vi "Add cod na fila.vi"(2 "error in (no error)":errorcluster, 3 "Queue in":refnum<queue>, 4 "Limite vertical":u32, 5 "Array Cluster in":T1(array[cluster])) -> (0 "error out":errorcluster, 1 "Array Cluster out":T1(array[cluster]))   [LabVIEW 2020]
uses:
  Type Defs/Cluster de envio.ctl
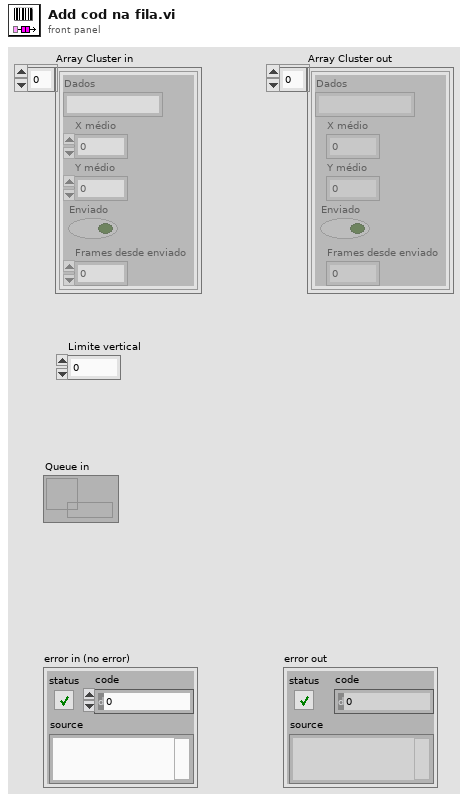
[diagram p1: front panel]
types:
  T1 = cluster{"Dados":string, "X médio":dbl, "Y médio":dbl, "Enviado":bool, "Frames desde enviado":dbl}[]
  T2 = typedef "Cluster de envio.ctl" = cluster{"Código de barras":string, "Quantidade":i32, "Data/Hora":timestamp}
  T3 = cluster{"Dados":string, "X médio":dbl, "Y médio":dbl, "Enviado":bool, "Frames desde enviado":dbl}
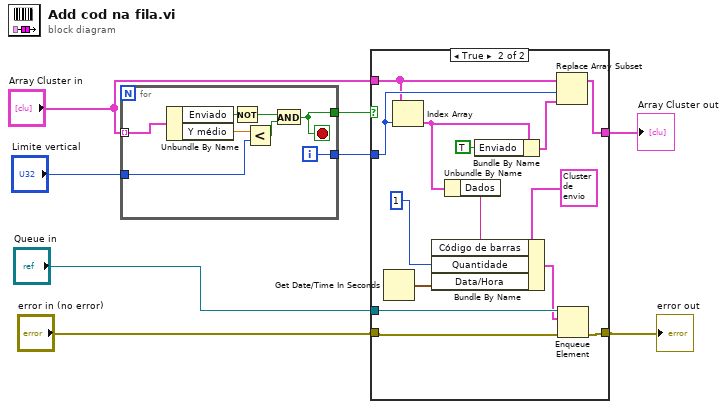
[diagram p0: block diagram]
diagram:
  n1 = for {
    tunnel: "Array Cluster in" -> [w16] mode=indexing
    tunnel: [w14] -> w2
    tunnel: [w10] -> w3
    tunnel: "Limite vertical" -> [w9]
    i -> [w14]
    stop <- w10 stop-if-true
    n2 = Unbundle By Name(w16) -> ("Enviado"=w12:bool, "Y médio"=w15:dbl)
    n3 = Not(x=w12) -> (.not. x?=w13:bool)
    n4 = Less?(x=w15, y=w9) -> (x < y?=w11:bool)
    n5 = And(x=w13, y=w11) -> (x .and. y?=w10:bool)
  }
  n6 = case shown="True" w3 {
    tunnel: "Array Cluster in" -> [w18 w23]
    tunnel: [w18 w25] -> w1
    tunnel: w2 -> [_ w24]
    tunnel: "Queue in" -> [_ w32]
    tunnel: "error in (no error)" -> [w17 w31]
    tunnel: [w17 w26] -> w6
    frame False {
    }
    frame True {
      n7 = Get Date/Time In Seconds() -> (seconds since 1Jan1904=w27:timestamp)
      n8 = Index Array(array=w23, index=w24) -> (element=w21:T3)
      n9 = Unbundle By Name(w21) -> ("Dados"=w22:string)
      n10 = Bundle By Name(cluster=T2 {"Código de barras"="", "Quantidade"=0, "Data/Hora"=timestamp(0 s since 1904-01-01)}, "Código de barras"=w22, "Quantidade"=1, "Data/Hora"=w27) -> (w29:T2)
      n11 = Bundle By Name(cluster=w21, "Enviado"=TRUE) -> (w20:T3)
      n12 = Replace Array Subset(array=w23, new element=w20, index=w24) -> (w25:T1)
      n13 = Enqueue Element(queue=w32, element=w29, error in (no error)=w31) -> (error out=w26:errorcluster)  [unwired: 1 in, 2 out]
    }
  }
  "error out" <- w6
  "Array Cluster out" <- w1
